vi "TrianglesRotate.vi"(10 "Rotation":T1, 11 "TrianglesIn":T2[](array[typedef])) -> (3 "TrianglesOut":T2[](array[typedef]))   [LabVIEW 2014]
uses:
  TypeDefs/TriangleFace.ctl
  TypeDefs/Point3D.ctl
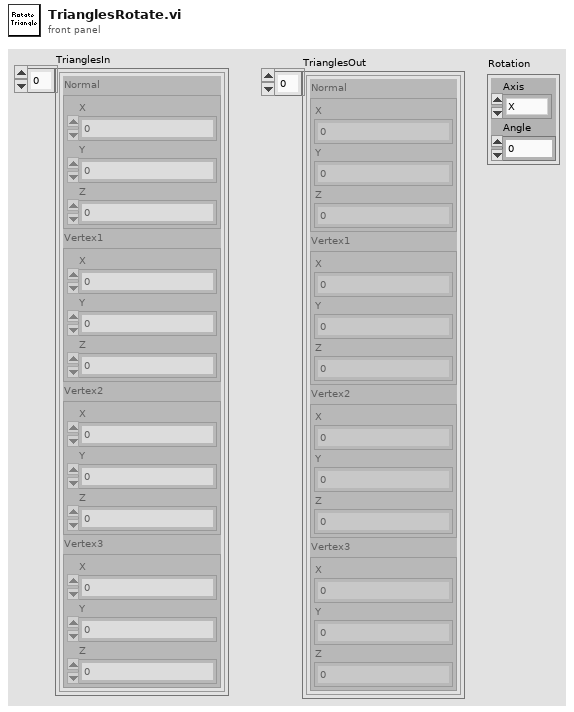
[diagram p1: front panel]
types:
  T1 = cluster{"Axis":enum16{"X", "Y", "Z"}, "Angle":sgl}
  T2 = typedef "TriangleFace.ctl" = cluster{"Normal":T3, "Vertex1":T3, "Vertex2":T3, "Vertex3":T3}
  T3 = typedef "Point3D.ctl" = cluster{"X":sgl, "Y":sgl, "Z":sgl}
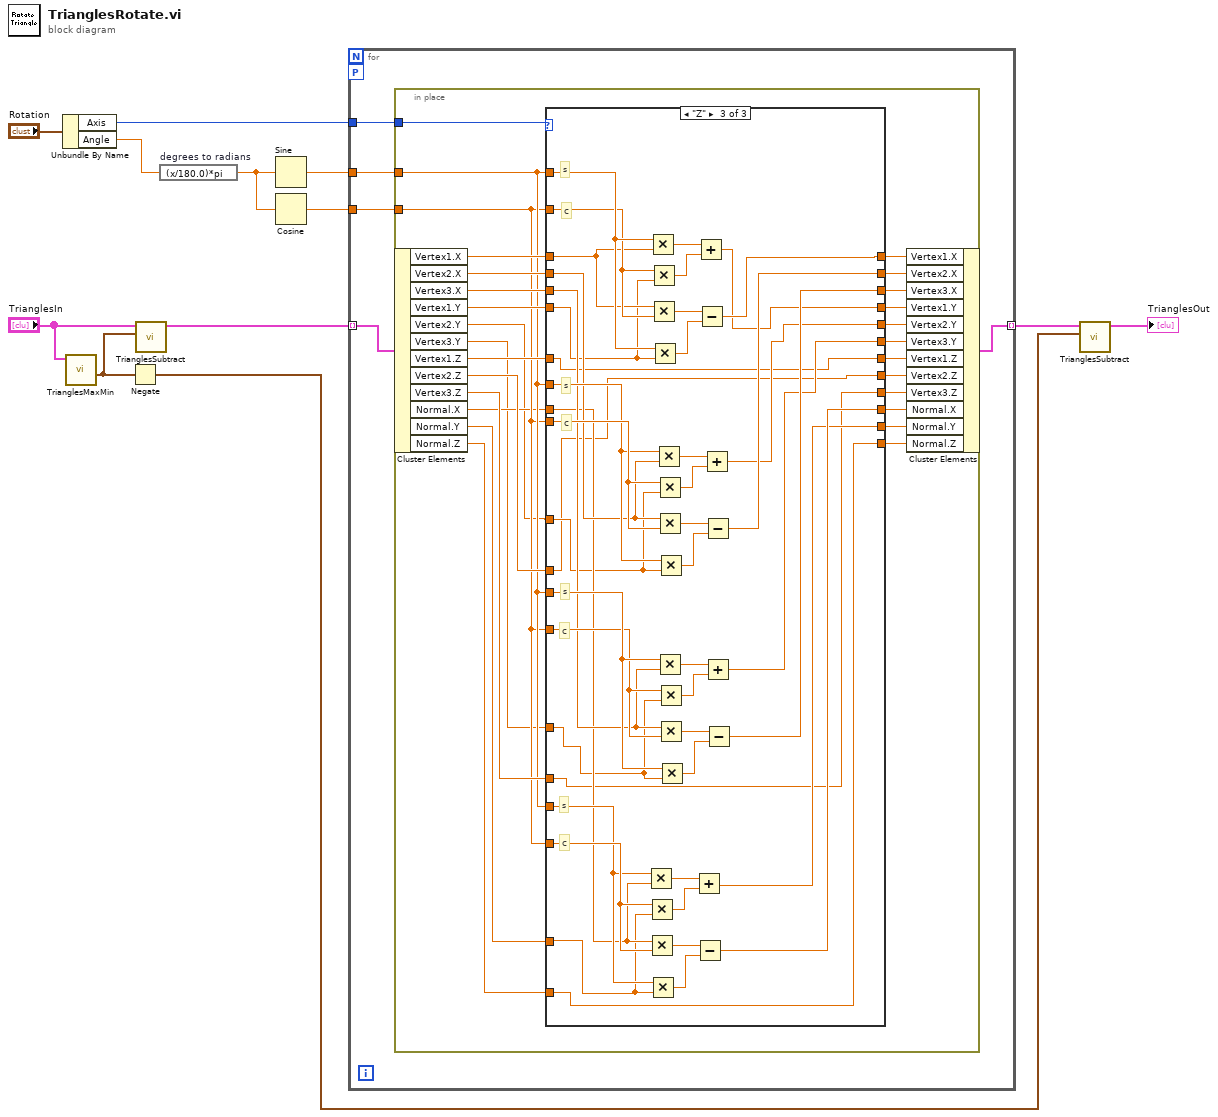
[diagram p0: block diagram]
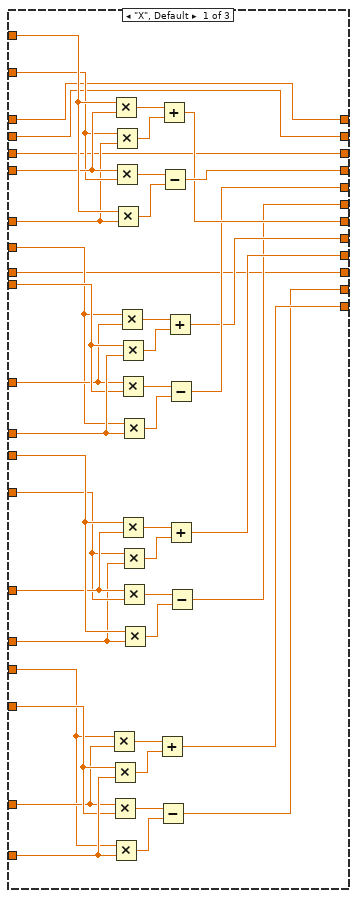
[diagram p2: hidden frame]
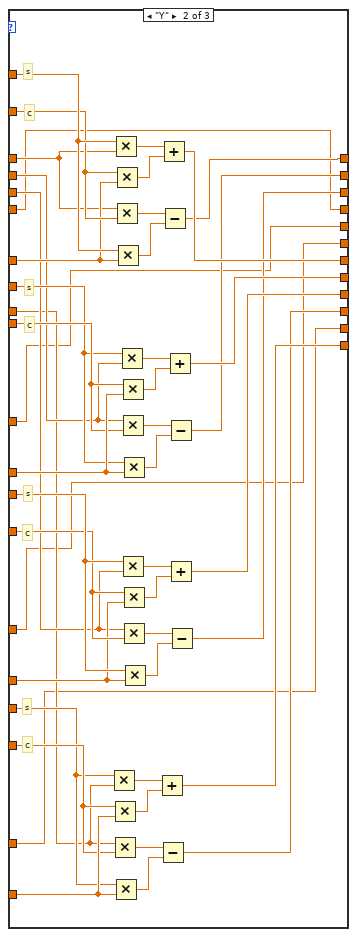
[diagram p3: hidden frame]
diagram:
  n1 = Unbundle By Name("Rotation") -> ("Axis"=w2:enum16{"X", "Y", "Z"}, "Angle"=w1:sgl)
  n2 = call "TrianglesMaxMin.vi"("Triangles"="TrianglesIn") -> ("Center"=w6:T3)  [unwired: 8 in, 2 out]
  n3 = Negate(x=w6) -> (-x=w5:T3)
  n4 = call "TrianglesSubtract.vi"("Point3D"=w6, "TrianglesIn"="TrianglesIn") -> ("TrianglesOut"=w11:T2[])  [unwired: 9 in]
  n5 = expression code="(x/180.0)*pi" "degrees to radians"(w1) -> (w10:sgl)
  n6 = Sine(x=w10) -> (sin(x)=w9:sgl)
  n7 = Cosine(x=w10) -> (cos(x)=w8:sgl)
  n8 = for {
    tunnel: w11 -> [w17] mode=indexing
    tunnel: [w16] -> w7 mode=indexing
    workers-P: _ -> [_]
    tunnel: w2 -> [w15]
    tunnel: w9 -> [w14]
    tunnel: w8 -> [w13]
    n9 = in-place {
      in-place-border: w15 -> [w44]
      in-place-border: w14 -> [w27]
      in-place-border: w13 -> [w26]
      n10 = in-place-cluster #1(w17) -> ("Vertex1.X"=w33:sgl, "Vertex2.X"=w32:sgl, "Vertex3.X"=w31:sgl, "Vertex1.Y"=w43:sgl, "Vertex2.Y"=w19:sgl, "Vertex3.Y"=w18:sgl, "Vertex1.Z"=w42:sgl, "Vertex2.Z"=w39:sgl, "Vertex3.Z"=w36:sgl, "Normal.X"=w22:sgl, "Normal.Y"=w25:sgl, "Normal.Z"=w24:sgl)
      n11 = case shown="\"Z\"" w44 {
        tunnel: w27 -> [w83 w128 w172]
        tunnel: w26 -> [w81 w127 w171]
        tunnel: w43 -> [w82 w92 w144]
        tunnel: w42 -> [w80 w126 w135]
        tunnel: [w86 w92 w138] -> w41
        tunnel: [w79 w125 w135] -> w40
        tunnel: w27 -> [w75 w122 w169]
        tunnel: w26 -> [w77 w123 w170]
        tunnel: w19 -> [w76 w91 w143]
        tunnel: w39 -> [w78 w124 w134]
        tunnel: [w59 w91 w137] -> w38
        tunnel: [w58 w110 w134] -> w37
        tunnel: w27 -> [w66 w113 w160]
        tunnel: w26 -> [w64 w112 w159]
        tunnel: w18 -> [w65 w90 w141]
        tunnel: w36 -> [w63 w111 w133]
        tunnel: [w56 w90 w136] -> w35
        tunnel: [w57 w109 w133] -> w34
        tunnel: w33 -> [w62 w100 w152]
        tunnel: w32 -> [w61 w98 w150]
        tunnel: w31 -> [w60 w96 w148]
        tunnel: [w62 w99 w151] -> w30
        tunnel: [w61 w97 w149] -> w29
        tunnel: [w60 w95 w147] -> w28
        tunnel: w27 -> [w52 w106 w157]
        tunnel: w26 -> [w54 w107 w158]
        tunnel: w25 -> [w53 w89 w142]
        tunnel: w24 -> [w55 w108 w139]
        tunnel: [w47 w93 w145] -> w23
        tunnel: w22 -> [w47 w94 w146]
        tunnel: [w46 w101 w139] -> w21
        tunnel: [w45 w89 w140] -> w20
        frame "X", Default {
          n12 = Multiply(x=w52, y=w53) -> (x*y=w51:sgl)
          n13 = Multiply(x=w54, y=w55) -> (x*y=w50:sgl)
          n14 = Multiply(x=w53, y=w54) -> (x*y=w48:sgl)
          n15 = Multiply(x=w83, y=w82) -> (x*y=w84:sgl)
          n16 = Multiply(x=w52, y=w55) -> (x*y=w49:sgl)
          n17 = Multiply(x=w81, y=w80) -> (x*y=w85:sgl)
          n18 = Multiply(x=w82, y=w81) -> (x*y=w88:sgl)
          n19 = Multiply(x=w83, y=w80) -> (x*y=w87:sgl)
          n20 = Multiply(x=w75, y=w76) -> (x*y=w74:sgl)
          n21 = Multiply(x=w77, y=w78) -> (x*y=w73:sgl)
          n22 = Multiply(x=w76, y=w77) -> (x*y=w71:sgl)
          n23 = Multiply(x=w66, y=w65) -> (x*y=w67:sgl)
          n24 = Multiply(x=w75, y=w78) -> (x*y=w72:sgl)
          n25 = Multiply(x=w64, y=w63) -> (x*y=w68:sgl)
          n26 = Multiply(x=w65, y=w64) -> (x*y=w70:sgl)
          n27 = Multiply(x=w66, y=w63) -> (x*y=w69:sgl)
          n28 = Add(x=w51, y=w50) -> (x+y=w46:sgl)
          n29 = Subtract(x=w48, y=w49) -> (x-y=w45:sgl)
          n30 = Add(x=w84, y=w85) -> (x+y=w79:sgl)
          n31 = Subtract(x=w88, y=w87) -> (x-y=w86:sgl)
          n32 = Add(x=w74, y=w73) -> (x+y=w58:sgl)
          n33 = Subtract(x=w71, y=w72) -> (x-y=w59:sgl)
          n34 = Add(x=w67, y=w68) -> (x+y=w57:sgl)
          n35 = Subtract(x=w70, y=w69) -> (x-y=w56:sgl)
        }
        frame "Y" {
          # "c"
          # "c"
          # "c"
          # "c"
          # "s"
          # "s"
          # "s"
          # "s"
          n36 = Multiply(x=w106, y=w94) -> (x*y=w105:sgl)
          n37 = Multiply(x=w107, y=w108) -> (x*y=w104:sgl)
          n38 = Multiply(x=w94, y=w107) -> (x*y=w102:sgl)
          n39 = Multiply(x=w128, y=w100) -> (x*y=w129:sgl)
          n40 = Multiply(x=w106, y=w108) -> (x*y=w103:sgl)
          n41 = Multiply(x=w127, y=w126) -> (x*y=w130:sgl)
          n42 = Multiply(x=w100, y=w127) -> (x*y=w132:sgl)
          n43 = Multiply(x=w128, y=w126) -> (x*y=w131:sgl)
          n44 = Multiply(x=w122, y=w98) -> (x*y=w121:sgl)
          n45 = Multiply(x=w123, y=w124) -> (x*y=w120:sgl)
          n46 = Multiply(x=w98, y=w123) -> (x*y=w118:sgl)
          n47 = Multiply(x=w113, y=w96) -> (x*y=w114:sgl)
          n48 = Multiply(x=w122, y=w124) -> (x*y=w119:sgl)
          n49 = Multiply(x=w112, y=w111) -> (x*y=w115:sgl)
          n50 = Multiply(x=w96, y=w112) -> (x*y=w117:sgl)
          n51 = Multiply(x=w113, y=w111) -> (x*y=w116:sgl)
          n52 = Add(x=w105, y=w104) -> (x+y=w101:sgl)
          n53 = Subtract(x=w102, y=w103) -> (x-y=w93:sgl)
          n54 = Add(x=w129, y=w130) -> (x+y=w125:sgl)
          n55 = Subtract(x=w132, y=w131) -> (x-y=w99:sgl)
          n56 = Add(x=w121, y=w120) -> (x+y=w110:sgl)
          n57 = Subtract(x=w118, y=w119) -> (x-y=w97:sgl)
          n58 = Add(x=w114, y=w115) -> (x+y=w109:sgl)
          n59 = Subtract(x=w117, y=w116) -> (x-y=w95:sgl)
        }
        frame "Z" {
          # "c"
          # "c"
          # "c"
          # "c"
          # "s"
          # "s"
          # "s"
          # "s"
          n60 = Multiply(x=w157, y=w146) -> (x*y=w156:sgl)
          n61 = Multiply(x=w158, y=w142) -> (x*y=w155:sgl)
          n62 = Multiply(x=w146, y=w158) -> (x*y=w153:sgl)
          n63 = Multiply(x=w172, y=w152) -> (x*y=w173:sgl)
          n64 = Multiply(x=w157, y=w142) -> (x*y=w154:sgl)
          n65 = Multiply(x=w171, y=w144) -> (x*y=w174:sgl)
          n66 = Multiply(x=w152, y=w171) -> (x*y=w176:sgl)
          n67 = Multiply(x=w172, y=w144) -> (x*y=w175:sgl)
          n68 = Multiply(x=w169, y=w150) -> (x*y=w168:sgl)
          n69 = Multiply(x=w170, y=w143) -> (x*y=w167:sgl)
          n70 = Multiply(x=w150, y=w170) -> (x*y=w165:sgl)
          n71 = Multiply(x=w160, y=w148) -> (x*y=w161:sgl)
          n72 = Multiply(x=w169, y=w143) -> (x*y=w166:sgl)
          n73 = Multiply(x=w159, y=w141) -> (x*y=w162:sgl)
          n74 = Multiply(x=w148, y=w159) -> (x*y=w164:sgl)
          n75 = Multiply(x=w160, y=w141) -> (x*y=w163:sgl)
          n76 = Add(x=w156, y=w155) -> (x+y=w140:sgl)
          n77 = Subtract(x=w153, y=w154) -> (x-y=w145:sgl)
          n78 = Add(x=w173, y=w174) -> (x+y=w138:sgl)
          n79 = Subtract(x=w176, y=w175) -> (x-y=w151:sgl)
          n80 = Add(x=w168, y=w167) -> (x+y=w137:sgl)
          n81 = Subtract(x=w165, y=w166) -> (x-y=w149:sgl)
          n82 = Add(x=w161, y=w162) -> (x+y=w136:sgl)
          n83 = Subtract(x=w164, y=w163) -> (x-y=w147:sgl)
        }
      }
      n84 = in-place-cluster #1("Vertex1.X"=w30, "Vertex2.X"=w29, "Vertex3.X"=w28, "Vertex1.Y"=w41, "Vertex2.Y"=w38, "Vertex3.Y"=w35, "Vertex1.Z"=w40, "Vertex2.Z"=w37, "Vertex3.Z"=w34, "Normal.X"=w23, "Normal.Y"=w20, "Normal.Z"=w21) -> (w16:T2)
    }
  }
  n85 = call "TrianglesSubtract.vi"("Point3D"=w5, "TrianglesIn"=w7) -> ("TrianglesOut"=→"TrianglesOut":T2[])  [unwired: 9 in]
